vi "G4BaseTemplate_Singleton_4x4x4_CleanUp.vi"(8 "error in (no error)":errorcluster) -> (0 "error out":errorcluster)   [LabVIEW 2016, in "G4BaseTemplate_Singleton_4x4x4.lvclass"]
uses:
  <resource>/Framework/Providers/Open_GDS/ClassProviders/Provider_EndevoGOOP400/Templates/G4BaseTemplate_Singleton_4x4x4/G4BaseTemplate_Singleton_4x4x4.lvclass
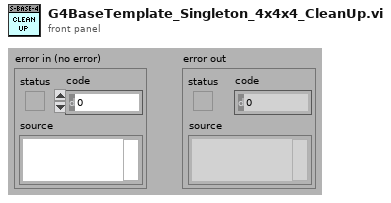
[diagram p1: front panel]
types:
  T1 = typedef "G4BaseTemplate_Singleton_4x4x4.lvclass/ObjectAttributes.ctl" = cluster{"Attribute1":dbl}
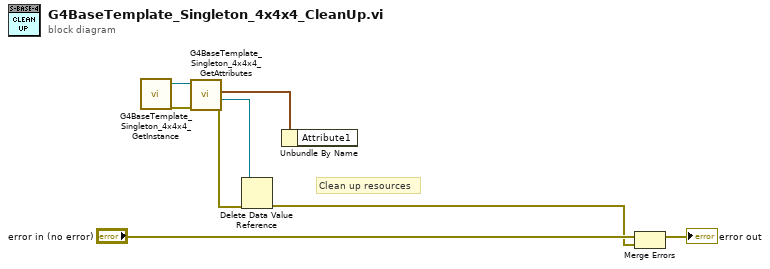
[diagram p0: block diagram]
diagram:
  # "Clean up resources"
  n1 = call <resource>:"G4BaseTemplate_Singleton_4x4x4_GetInstance.vi"() -> ("error out"=w6:errorcluster, "reference out"=w5:refnum<class "G4BaseTemplate_Singleton_4x4x4.lvclass">)  [unwired: 7 in, 3 out]
  n2 = call <resource>:"G4BaseTemplate_Singleton_4x4x4_GetAttributes.vi"("error in (no error)"=w6, "reference in"=w5) -> ("error out"=w4:errorcluster, "DataRef"=w3:refnum<data-value>, "Data"=w7:T1)  [unwired: 6 in, 1 out]
  n3 = Delete Data Value Reference(data value reference=w3, error in=w4) -> (error out=w1:errorcluster)  [unwired: 1 out]
  n4 = Unbundle By Name(w7) -> ()  [unwired: 1 out]
  n5 = Merge Errors("error in (no error)", w1) -> (→"error out":errorcluster)
